vi "_Predefined_SuperUser.vi"() -> (3 "SuperUsers":T1[](array[typedef]))   [LabVIEW 2017, in "Login-UI.lvlib"]
uses:
  Login-UI.lvlib
  User-Info.ctl
  User-Role.ctl
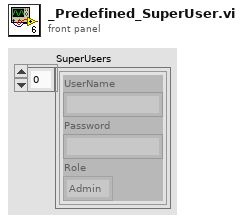
[diagram p1: front panel]
types:
  T1 = typedef "Login-UI.lvlib/User-Info.ctl" = cluster{"UserName":string, "Password":string, "Role":T2}
  T2 = typedef "Login-UI.lvlib/User-Role.ctl" = enum16{"INVALID", "Operator", "Engineer", "Admin"}
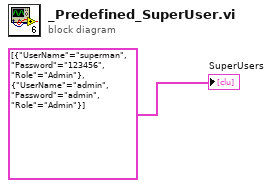
[diagram p0: block diagram]
diagram:
  "SuperUsers" <- T1[] [{"UserName"="superman", "Password"="123456", "Role"=enum."Admin"}, {"UserName"="admin", "Password"="admin", "Role"=enum."Admin"}] ("Array")
